vi "Variant to Formatted String v2.vi"(6 "Tokens to keep (all)":bool[](array[boolean]), 8 "error in (no error)":errorcluster, 11 "Anything":variant) -> (0 "error out":errorcluster, 3 "String":string)   [LabVIEW 2021, in "Variant.lvlib"]
doc: "Gets the text of the variant"
uses:
  Variant.lvlib
  dd5c9caf-7c87-4227-896a-f6a249a2d77c.vi
  <vilib>/JDP Science/JSONtext/Variant to JSON Text.vi
  <vilib>/JDP Science/JSONtext/LVClass Serializer/JSONtext LVClass Serializer.lvclass
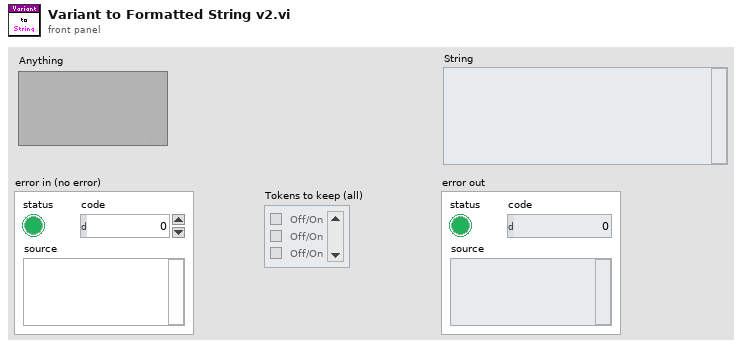
[diagram p1: front panel]
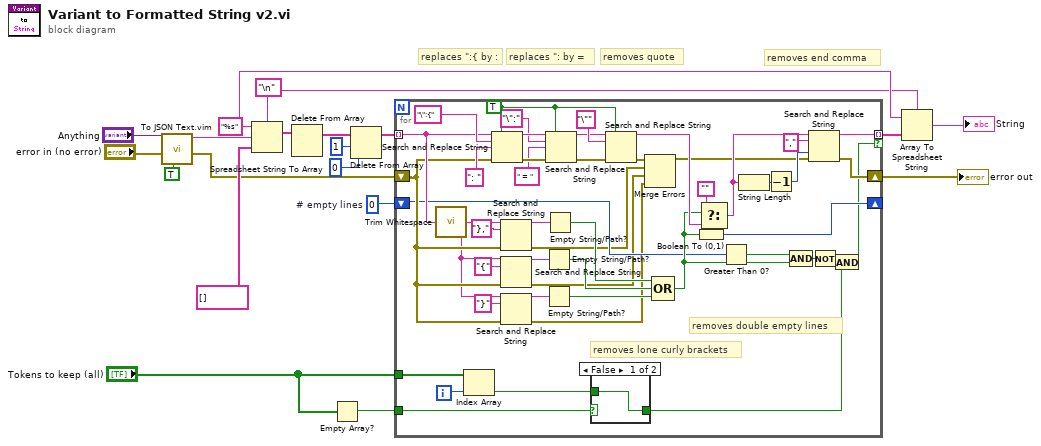
[diagram p0: block diagram]
diagram:
  w1 = 0  # # empty lines
  w8 = "%s" ("format string")
  w7 = "\n" ("delimiter (Tab)")
  # "replaces \":{ by :"
  # "removes end comma"
  # "removes quote"
  # "replaces \": by ="
  n1 = call "To JSON Text.vim"("Pretty Print?"=TRUE, "error in (no error)"="error in (no error)", "Anything"="Anything") -> ("error out"=w5:errorcluster, "<JSON>"=w16:string)  [unwired: 7 in]
  n2 = Spreadsheet String To Array(delimiter (Tab)=w7, format string=w8, spreadsheet string=w16, array type (2D Dbl)=string[] [] ("<JSON>")) -> (array=w14:string[])
  n3 = Delete From Array(array=w14) -> (array with subset deleted=w13:string[])  [unwired: 2 in, 1 out]
  n4 = Empty Array?(array="Tokens to keep (all)") -> (empty?=w2:bool)
  n5 = Delete From Array(array=w13, length=1, index=0) -> (array with subset deleted=w10:string[])  [unwired: 1 out]
  n6 = for {
    tunnel: w10 -> [w54] mode=indexing
    tunnel: [w34] -> w9 mode=indexing if=w21
    shift-right: [w28] -> w4
    shift-left: w5 -> [w43]
    tunnel: "Tokens to keep (all)" -> [w64]
    tunnel: w2 -> [w62]
    shift-right: [w38] -> _
    shift-left: w1 -> [w37]
    i -> [w63]
    w56 = TRUE ("replace all? (F)")
    # "removes lone curly brackets"
    # "removes double empty lines"
    n7 = call <vilib>:"Trim Whitespace.vi"("string"=w54) -> ("trimmed string"=w41:string)  [unwired: 1 in]
    n8 = Index Array(array=w64, index=w63) -> (element=w61:bool)
    n9 = Search and Replace String(replace all?=w56, input string=w54, search string="\":{", replace string=": " ("replace string (\"\")"), error in=w43) -> (result string=w60:string, error out=w57:errorcluster)  [unwired: 3 in, 2 out]
    n10 = Search and Replace String(input string=w41, search string="},", error in=w43) -> (result string=w48:string, error out=w26:errorcluster)  [unwired: 5 in, 2 out]
    n11 = Search and Replace String(input string=w41, search string="{", error in=w43) -> (result string=w49:string, error out=w25:errorcluster)  [unwired: 5 in, 2 out]
    n12 = Search and Replace String(input string=w41, search string="}", error in=w43) -> (result string=w44:string, error out=w24:errorcluster)  [unwired: 5 in, 2 out]
    n13 = Empty String/Path?(string/path=w49) -> (empty?=w47:bool)
    n14 = Empty String/Path?(string/path=w44) -> (empty?=w42:bool)
    n15 = Empty String/Path?(string/path=w48) -> (empty?=w52:bool)
    n16 = Search and Replace String(replace all?=w56, input string=w60, search string="\":", replace string=" = " ("replace string (\"\")"), error in=w57) -> (result string=w23:string, error out=w22:errorcluster)  [unwired: 3 in, 2 out]
    n17 = case shown="False" w62 {
      selector: w62 -> [_ w68]
      tunnel: [w67 w68] -> w20
      tunnel: w61 -> [w67 _]
      frame False {
      }
      frame True {
      }
    }
    n18 = Search and Replace String(replace all?=w56, input string=w23, search string="\"", error in=w22) -> (result string=w51:string, error out=w32:errorcluster)  [unwired: 4 in, 2 out]
    n19 = Merge Errors(w32, w26, w25, w24) -> (w27:errorcluster)
    n20 = Compound Arithmetic op=OR(w52, w47, w42) -> (w39:bool)
    n21 = Boolean To (0,1)(Boolean=w39) -> (0, 1=w38:i16)
    n22 = Select(t="", s=w39, f=w51) -> (s? t:f=w31:string)
    n23 = Greater Than 0?(x=w37) -> (x > 0?=w40:bool)
    n24 = String Length(string=w31) -> (length=w30:i32)
    n25 = Decrement(x=w30) -> (x-1=w29:i32)
    n26 = Compound Arithmetic op=AND(w40, w39) -> (w36:bool)
    n27 = Search and Replace String(input string=w31, search string=",", offset=w29, error in=w27) -> (result string=w34:string, error out=w28:errorcluster)  [unwired: 4 in, 2 out]
    n28 = Not(x=w36) -> (.not. x?=w35:bool)
    n29 = And(x=w35, y=w20) -> (x .and. y?=w21:bool)
  }
  "error out" <- w4
  n30 = Array To Spreadsheet String(delimiter (Tab)=w7, array=w9, 3:w8) -> (spreadsheet string=→"String":string)
